vi "Processes Launcher.vi"(8 "Error In":errorcluster, 11 "Dashboard In":refnum<class "Dashboard.lvclass">) -> (0 "Error Out":errorcluster, 3 "Dashboard Out":refnum<class "Dashboard.lvclass">)   [LabVIEW 2019, in "Dashboard.lvclass"]
uses:
  Dashboard.lvclass
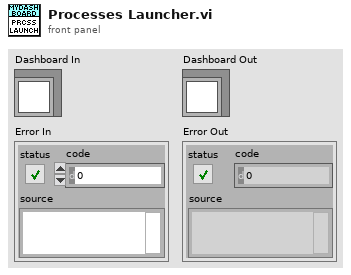
[diagram p1: front panel]
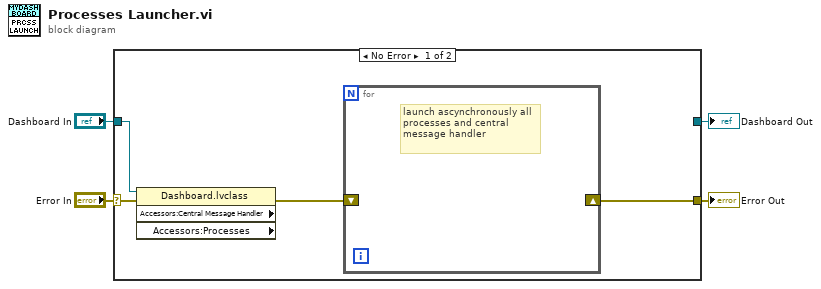
[diagram p0: block diagram]
diagram:
  n1 = case shown="No Error" "Error In" {
    selector: "Error In" -> [w7 w9]
    tunnel: "Dashboard In" -> [w8 w10]
    tunnel: [_ w10] -> w1
    tunnel: [w5 w9] -> w2
    frame No Error {
      n2 = property class="Dashboard.lvclass" props=["Accessors:Central Message Handler", "Accessors:Processes"](reference=w8, error in=w7) -> (error out=w6:errorcluster)  [unwired: 3 out]
      n3 = for {
        shift-right: [_] -> w5
        shift-left: w6 -> [_]
        # "launch ascynchronously all processes and central message handler"
      }
    }
    frame Error {
    }
  }
  "Dashboard Out" <- w1
  "Error Out" <- w2
